vi "Process_LaserStatus.vi"(11 "Data":string) -> (3 "output cluster":T1)   [LabVIEW 2021]
uses:
  TypeDefs/laser_cabinet_status.ctl
panel:
  out "Humidity":sgl
  out "Isolator Temperature (C)":sgl
  out "OM2 Temperature (C)":sgl
  out "OM1 Temperature (C)":sgl
  out "Remote Controller Temperature (C)":sgl
  out "Dew Point":sgl
  out "PSU Temperature (C)":sgl
  out "Back Reflection (mV)":sgl
  out "Analog power control (mV)":sgl
  out "Peak Power (kW)":sgl
  out "Pulse Energy (mJ)":sgl
  out "Pulse Duration (ns)":u32
  out "Measured Power (W)":sgl
  out "Measured Frequency (kHz)":sgl
  out "Reserved1":u16
  out "Extended Status":u32
  out "Warnings":u32
  out "Status":u32
  out "Extended Alarms":u32
  out "System Alarms":u32
  out "Alarms":u32
  out "Main Status":u32
  out "Set Power (%)":sgl
  out "Average Power (W)":sgl
  out "Set Frequency (kHz)":sgl
  out "Set Mode Index":u16
  out "Installed Status":u32
  out "Version":u16
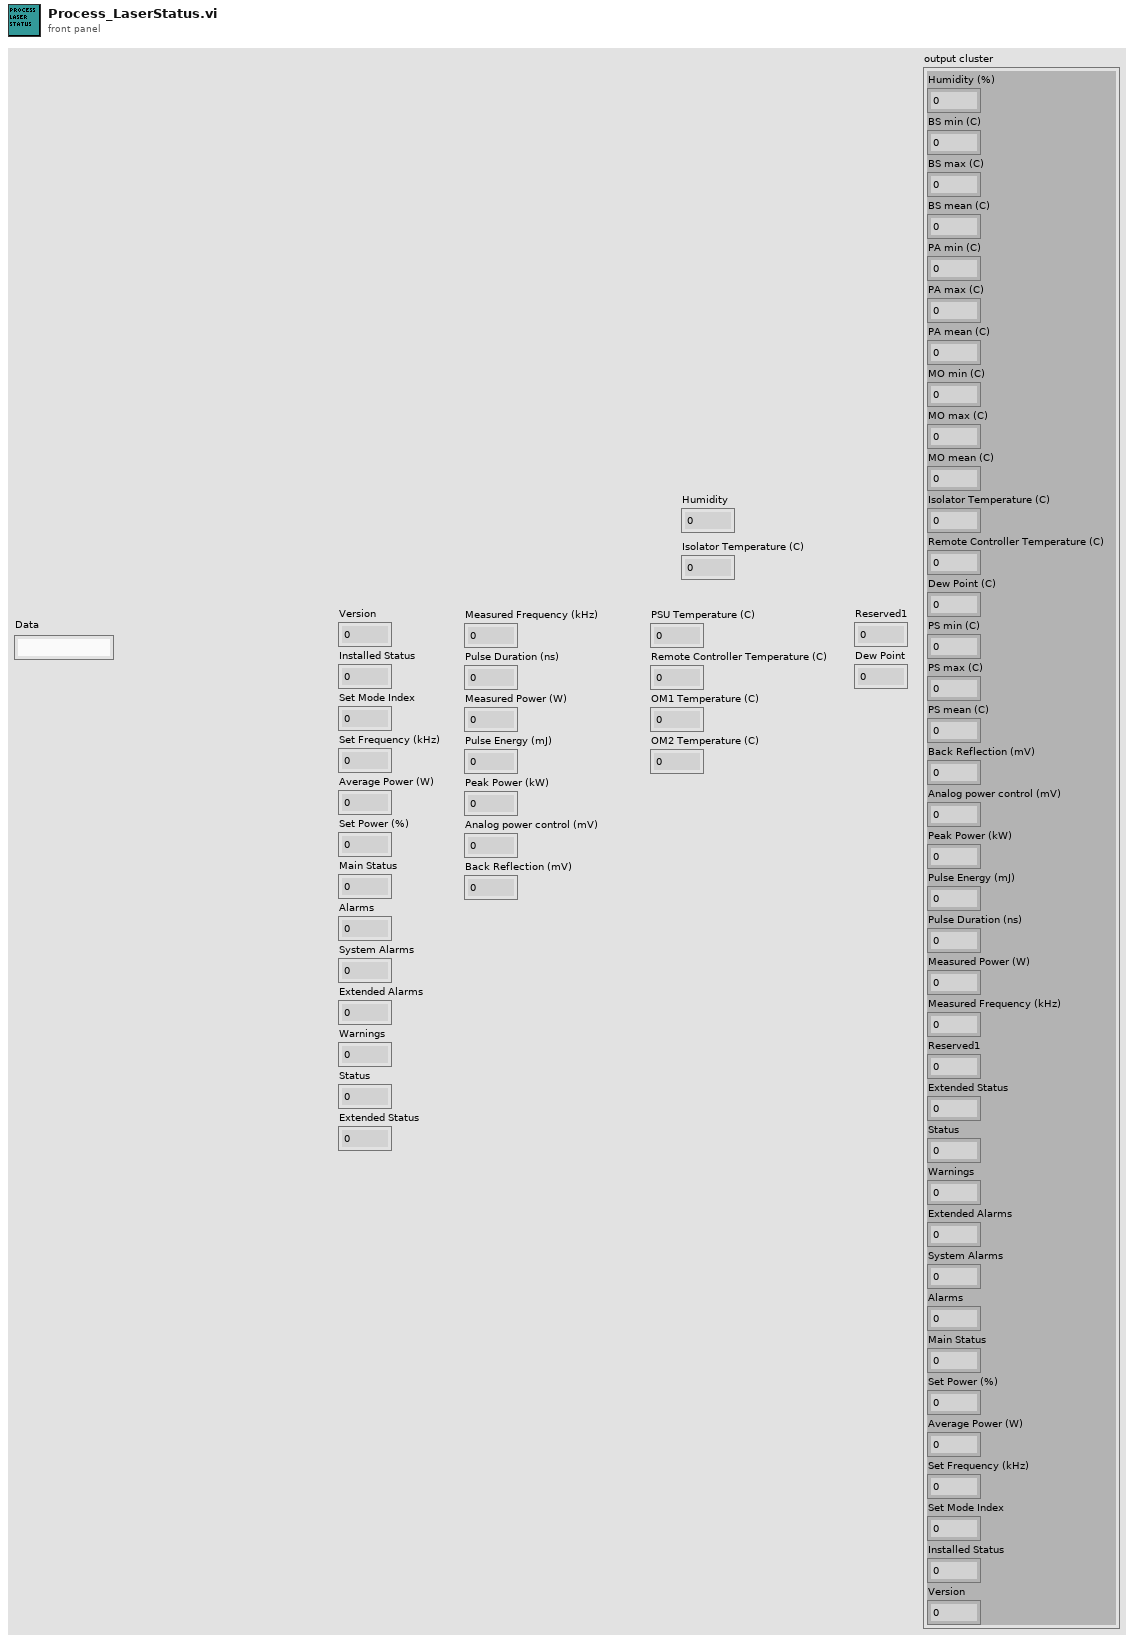
[diagram p1: front panel]
types:
  T1 = typedef "laser_cabinet_status.ctl" = cluster{"Version":u16, "Installed Status":u32, "Set Mode Index":u16, "Set Frequency (kHz)":sgl, "Average Power (W)":sgl, "Set Power (%)":sgl, "Main Status":u32, "Alarms":u32, "System Alarms":u32, "Extended Alarms":u32, "Warnings":u32, "Status":u32, "Extended Status":u32, "Reserved1":u16, "Measured Frequency (kHz)":sgl, "Pulse Duration (ns)":u32, "Measured Power (W)":sgl, "Pulse Energy (mJ)":sgl, "Peak Power (kW)":sgl, "Analog power control (mV)":sgl, "Back Reflection (mV)":sgl, "PS mean (C)":sgl, "PS max (C)":sgl, "PS min (C)":sgl, "Dew Point (C)":sgl, "Remote Controller Temperature (C)":sgl, "Isolator Temperature (C)":sgl, "MO mean (C)":sgl, "MO max (C)":sgl, "MO min (C)":sgl, "PA mean (C)":sgl, "PA max (C)":sgl, "PA min (C)":sgl, "BS mean (C)":sgl, "BS max (C)":sgl, "BS min (C)":sgl, "Humidity (%)":sgl}
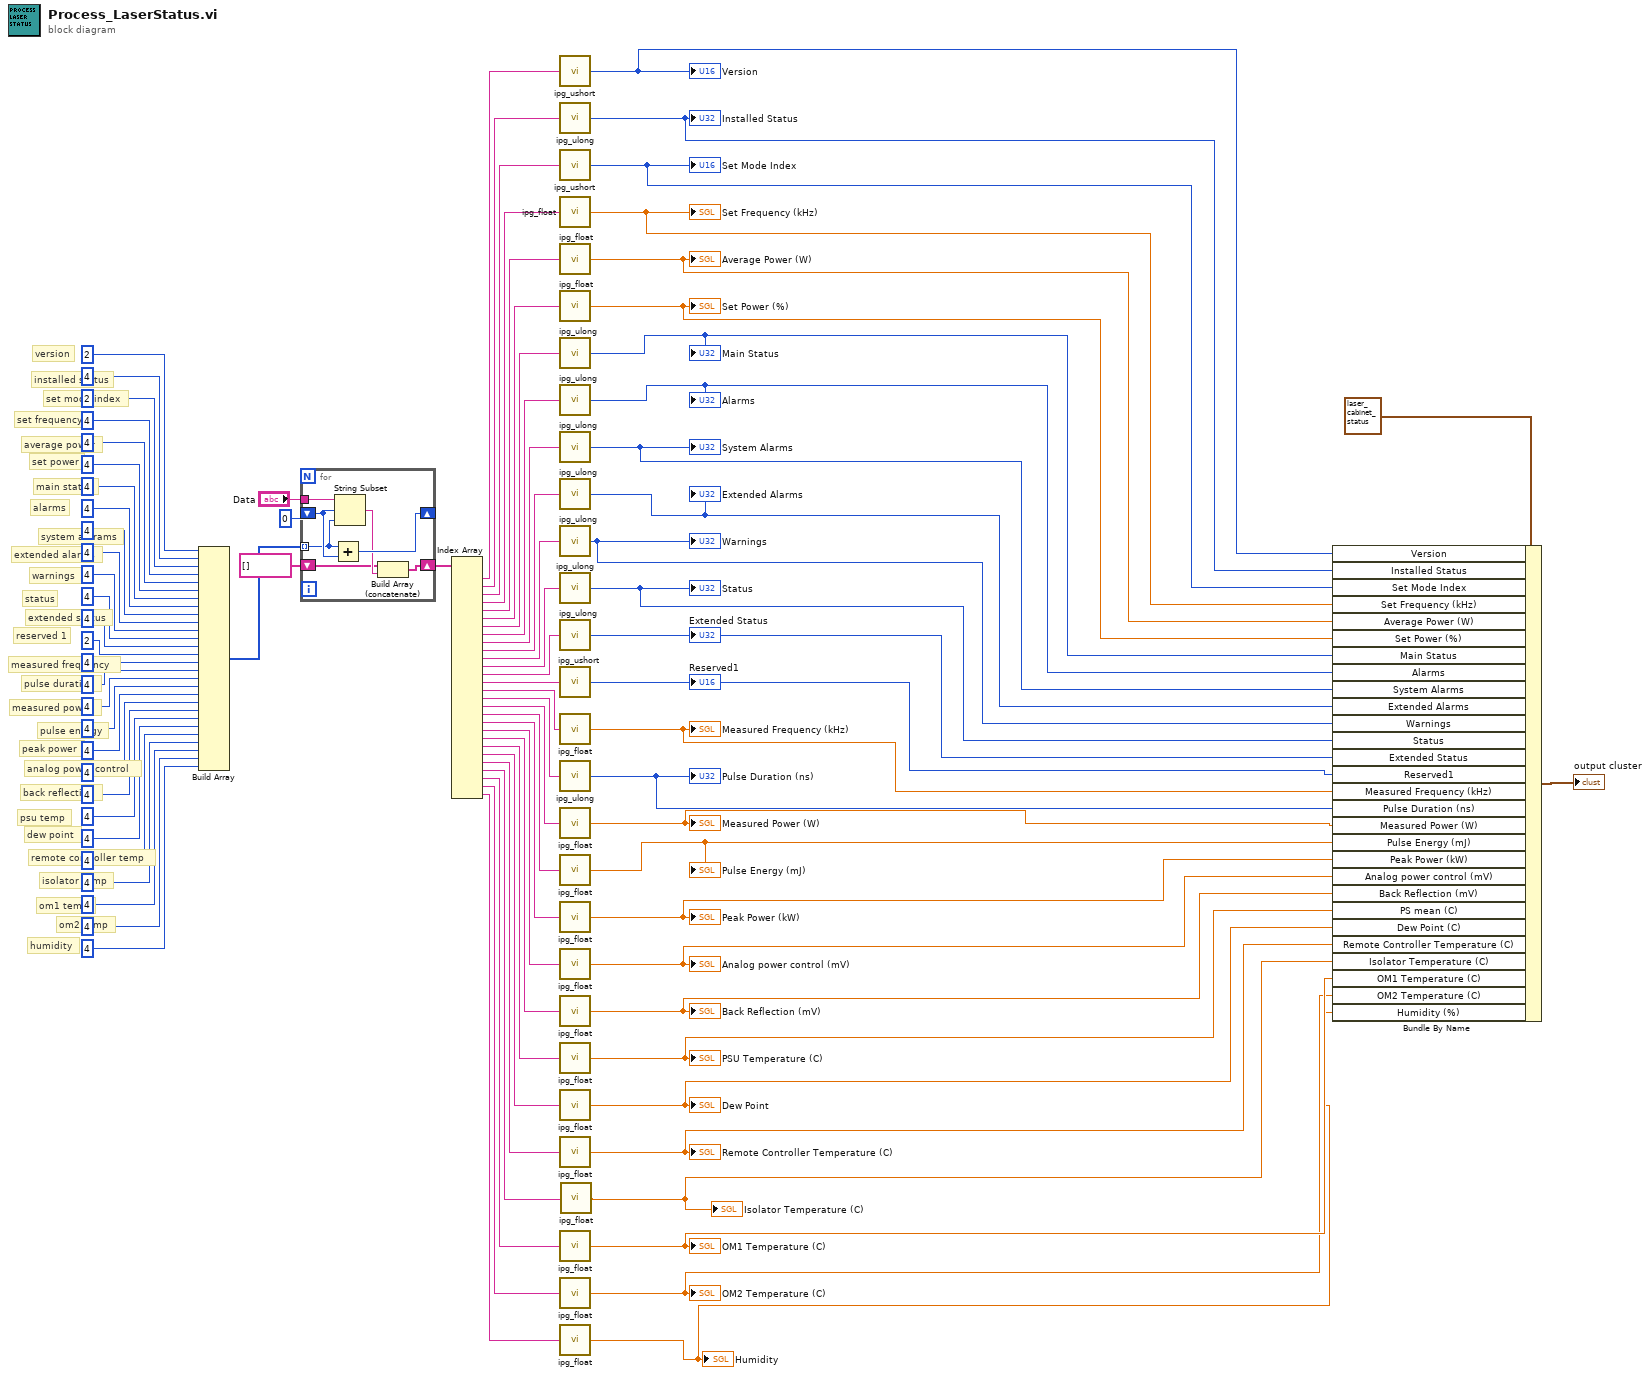
[diagram p0: block diagram]
diagram:
  # "humidity"
  # "om2 temp"
  # "om1 temp"
  # "isolator temp"
  # "remote controller temp"
  # "dew point"
  # "psu temp"
  # "back reflection"
  # "analog power control"
  # "peak power"
  # "pulse energy"
  # "measured power"
  # "pulse duration"
  # "measured frequency"
  # "reserved 1"
  # "extended status"
  # "status"
  # "warnings"
  # "extended alarms"
  # "system alarams"
  # "alarms"
  # "main status"
  # "set power"
  # "average power"
  # "set frequency"
  # "set mode index"
  # "installed status"
  # "version"
  n1 = Build Array(2, 4, 2, 4, 4, 4, 4, 4, 4, 4, 4, 4, 4, 2, 4, 4, 4, 4, 4, 4, 4, 4, 4, 4, 4, 4, 4, 4) -> (w63:i32[])
  n2 = for {
    tunnel: w63 -> [w95] mode=indexing
    shift-right: [w98] -> _
    shift-left: 0 -> [w96]
    tunnel: "Data" -> [w97]
    shift-right: [w93] -> w61
    shift-left: string[] [] -> [w92]
    n3 = Add(x=w95, y=w96) -> (x+y=w98:i32)
    n4 = String Subset(string=w97, offset (0)=w96, length (rest)=w95) -> (substring=w94:string)
    n5 = Build Array (concatenate)(w92, w94) -> (w93:string[])
  }
  n6 = Index Array(array=w61) -> (element #1=w60:string, element #2=w59:string, element #3=w58:string, element #4=w57:string, element #5=w56:string, element #6=w55:string, element #7=w54:string, element #8=w53:string, element #9=w52:string, element #10=w51:string, element #11=w50:string, element #12=w49:string, element #13=w48:string, element #14=w47:string, element #15=w46:string, element #16=w45:string, element #17=w44:string, element #18=w43:string, element #19=w42:string, element #20=w41:string, element #21=w40:string, element #22=w39:string, element #23=w10:string, element #24=w38:string, element #25=w8:string, element #26=w37:string, element #27=w36:string, element #28=w6:string)  [unwired: 28 in]
  n7 = call "ipg_ushort.vi"("String"=w60) -> ("Ushort"=w35:u16)
  "Version" <- w35
  n8 = call "ipg_ulong.vi"("String"=w59) -> ("Ulong"=w34:u32)
  "Installed Status" <- w34
  n9 = call "ipg_ushort.vi"("String"=w58) -> ("Ushort"=w33:u16)
  "Set Mode Index" <- w33
  n10 = call "ipg_float.vi"("String"=w57) -> ("Float"=w32:sgl)
  "Set Frequency (kHz)" <- w32
  n11 = call "ipg_float.vi"("String"=w56) -> ("Float"=w31:sgl)
  "Average Power (W)" <- w31
  n12 = call "ipg_float.vi"("String"=w55) -> ("Float"=w30:sgl)
  "Set Power (%)" <- w30
  n13 = call "ipg_ulong.vi"("String"=w54) -> ("Ulong"=w29:u32)
  "Main Status" <- w29
  n14 = call "ipg_ulong.vi"("String"=w53) -> ("Ulong"=w28:u32)
  "Alarms" <- w28
  n15 = call "ipg_ulong.vi"("String"=w52) -> ("Ulong"=w27:u32)
  "System Alarms" <- w27
  n16 = call "ipg_ulong.vi"("String"=w51) -> ("Ulong"=w26:u32)
  "Extended Alarms" <- w26
  n17 = call "ipg_ulong.vi"("String"=w50) -> ("Ulong"=w25:u32)
  "Warnings" <- w25
  n18 = call "ipg_ulong.vi"("String"=w49) -> ("Ulong"=w24:u32)
  "Status" <- w24
  n19 = call "ipg_ulong.vi"("String"=w48) -> ("Ulong"=w23:u32)
  "Extended Status" <- w23
  n20 = call "ipg_ushort.vi"("String"=w47) -> ("Ushort"=w22:u16)
  "Reserved1" <- w22
  n21 = call "ipg_float.vi"("String"=w46) -> ("Float"=w21:sgl)
  "Measured Frequency (kHz)" <- w21
  n22 = call "ipg_ulong.vi"("String"=w45) -> ("Ulong"=w14:u32)
  "Pulse Duration (ns)" <- w14
  n23 = call "ipg_float.vi"("String"=w44) -> ("Float"=w13:sgl)
  "Measured Power (W)" <- w13
  n24 = call "ipg_float.vi"("String"=w43) -> ("Float"=w20:sgl)
  "Pulse Energy (mJ)" <- w20
  n25 = call "ipg_float.vi"("String"=w42) -> ("Float"=w19:sgl)
  "Peak Power (kW)" <- w19
  n26 = call "ipg_float.vi"("String"=w41) -> ("Float"=w18:sgl)
  "Analog power control (mV)" <- w18
  n27 = call "ipg_float.vi"("String"=w40) -> ("Float"=w17:sgl)
  "Back Reflection (mV)" <- w17
  n28 = call "ipg_float.vi"("String"=w39) -> ("Float"=w16:sgl)
  "PSU Temperature (C)" <- w16
  n29 = call "ipg_float.vi"("String"=w10) -> ("Float"=w9:sgl)
  "Dew Point" <- w9
  n30 = call "ipg_float.vi"("String"=w38) -> ("Float"=w15:sgl)
  "Remote Controller Temperature (C)" <- w15
  n31 = call "ipg_float.vi"("String"=w37) -> ("Float"=w3:sgl)
  "OM1 Temperature (C)" <- w3
  n32 = call "ipg_float.vi"("String"=w36) -> ("Float"=w2:sgl)
  "OM2 Temperature (C)" <- w2
  n33 = call "ipg_float.vi"("String"=w6) -> ("Float"=w1:sgl)
  "Humidity" <- w1
  n34 = call "ipg_float.vi"("String"=w8) -> ("Float"=w7:sgl)
  "Isolator Temperature (C)" <- w7
  n35 = Bundle By Name(cluster=T1 {"Version"=0, "Installed Status"=0, "Set Mode Index"=0, "Set Frequency (kHz)"=0.0, "Average Power (W)"=0.0, "Set Power (%)"=0.0, "Main Status"=0, "Alarms"=0, "System Alarms"=0, "Extended Alarms"=0, "Warnings"=0, "Status"=0, "Extended Status"=0, "Reserved1"=0, "Measured Frequency (kHz)"=0.0, "Pulse Duration (ns)"=0, "Measured Power (W)"=0.0, "Pulse Energy (mJ)"=0.0, "Peak Power (kW)"=0.0, "Analog power control (mV)"=0.0, "Back Reflection (mV)"=0.0, "PS mean (C)"=0.0, "PS max (C)"=0.0, "PS min (C)"=0.0, "Dew Point (C)"=0.0, "Remote Controller Temperature (C)"=0.0, "Isolator Temperature (C)"=0.0, "MO mean (C)"=0.0, "MO max (C)"=0.0, "MO min (C)"=0.0, "PA mean (C)"=0.0, "PA max (C)"=0.0, "PA min (C)"=0.0, "BS mean (C)"=0.0, "BS max (C)"=0.0, "BS min (C)"=0.0, "Humidity (%)"=0.0} ("init_cluster"), "Version"=w35, "Installed Status"=w34, "Set Mode Index"=w33, "Set Frequency (kHz)"=w32, "Average Power (W)"=w31, "Set Power (%)"=w30, "Main Status"=w29, "Alarms"=w28, "System Alarms"=w27, "Extended Alarms"=w26, "Warnings"=w25, "Status"=w24, "Extended Status"=w23, "Reserved1"=w22, "Measured Frequency (kHz)"=w21, "Pulse Duration (ns)"=w14, "Measured Power (W)"=w13, "Pulse Energy (mJ)"=w20, "Peak Power (kW)"=w19, "Analog power control (mV)"=w18, "Back Reflection (mV)"=w17, "PS mean (C)"=w16, "Dew Point (C)"=w9, "Remote Controller Temperature (C)"=w15, "Isolator Temperature (C)"=w7, "OM1 Temperature (C)"=w3, "OM2 Temperature (C)"=w2, "Humidity (%)"=w1) -> (→"output cluster":T1)
